vi "Pinholes.vi"(4 "Current Threshold [nA]":dbl, 5 "settling\ndelay":i32) -> (1 "excluded channels":i32[](array[numeric]), 2 "Current [nA]":dbl[](array[numeric]), 3 "Flag":i32[](array[numeric]))   [LabVIEW 2018]
uses:
  general_VIs/globals/QC_MeasurementSetup.vi
  InstrControl/Switching/Switching.lvclass
  InstrControl/SupplyControl/SupplyControl.lvclass
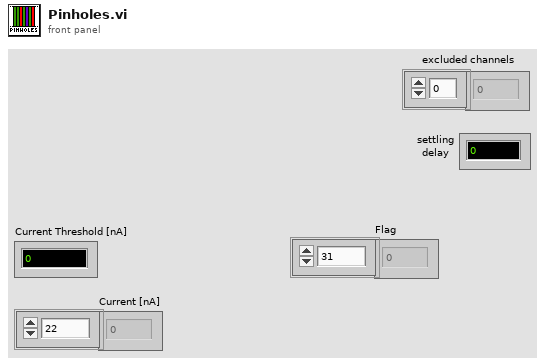
[diagram p1: front panel]
types:
  T1 = cluster{"Bias Supply":refnum<class "SupplyControl.lvclass">, "SMU":refnum<class "SupplyControl.lvclass">, "LCR":refnum<class "LCRControl.lvclass">, "Probe Card Channels":i32, "Bias Voltage [V]":dbl, "First strip":i32, "Last strip":i32, "Base Voltage [V]":dbl, "Base Ramp Step [V]":dbl, "Base Ramp Interval [ms]":u32, "High Voltage [V]":dbl, "High Ramp Step [V]":dbl, "High Ramp Interval [ms]":u32, "Single Needle":bool, "Temperature Readout":enum16{"Read Arduino", "Enter manually"}, "Arduino":refnum<class "ArduinoControl.lvclass">, "Fraction of good strips [%]":dbl, "ProbeStation":refnum<class "ProbeStationControl.lvclass">, "AC frequency [Hz]":i32, "Switching":refnum<class "Switching.lvclass">, "Matrix used?":bool, "Matrix X Channels":cluster{"Bias Supply / SMU LO":i32, "Bias Supply / SMU HI":i32, "CV Box LO":i32, "CV Box HI":i32, "CV Box LO IN":i32, "CV Box HI IN":i32, "Volt meter LO":i32, "Volt meter HI":i32, "Mux1 C1":i32, "Mux1 C2":i32, "Mux2 C1":i32, "Mux2 C2":i32}, "Pinholes Y/N":bool, "Capacitance Y/N":bool, "Resistance Y/N":bool}
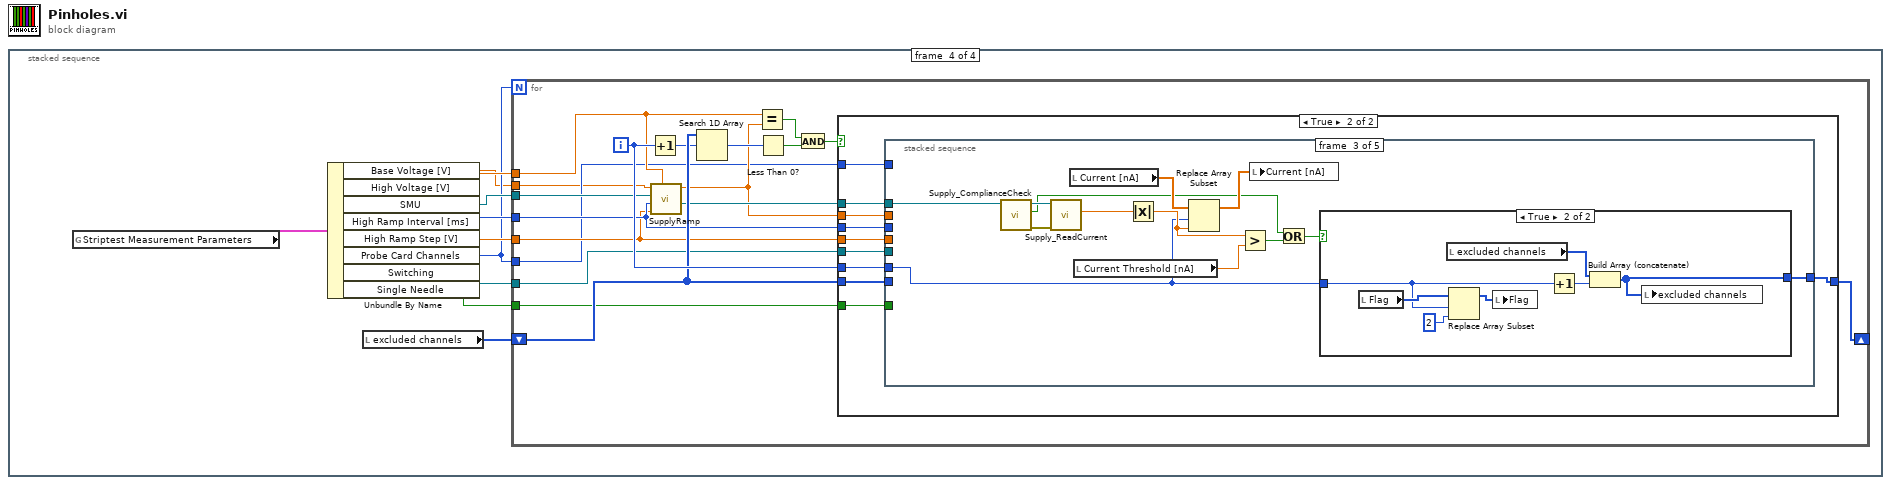
[diagram p0: block diagram]
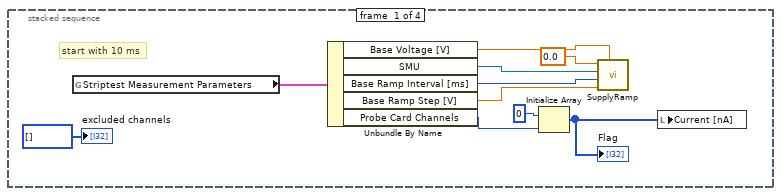
[diagram p2: hidden frame]
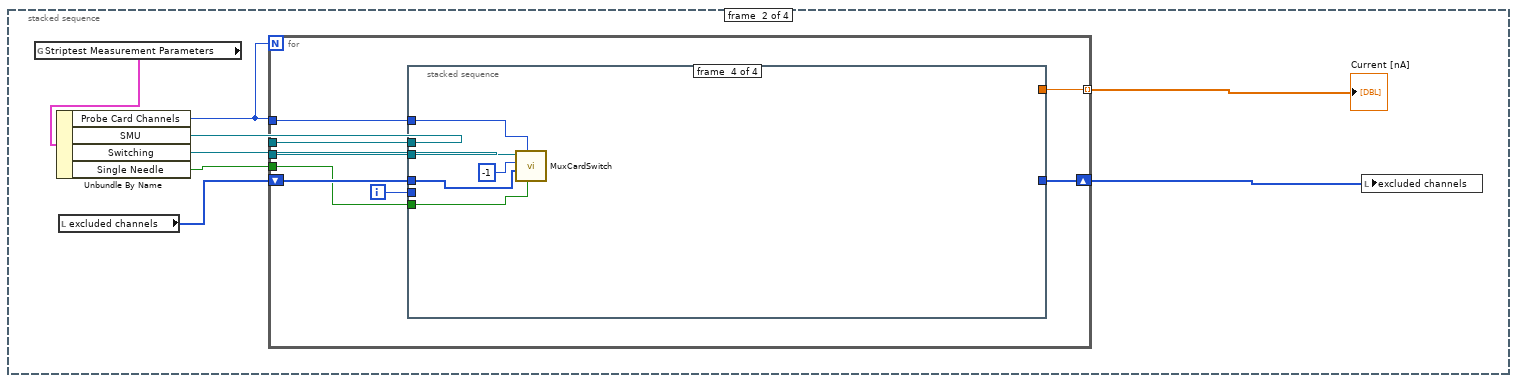
[diagram p3: hidden frame]
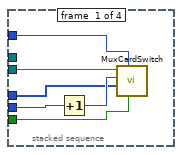
[diagram p4: hidden frame]
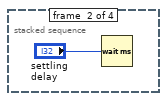
[diagram p5: hidden frame]
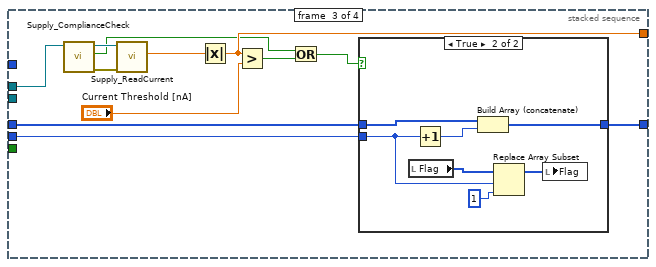
[diagram p6: hidden frame]
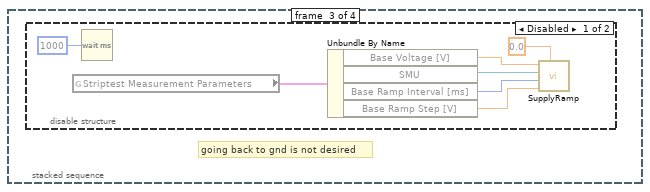
[diagram p8: hidden frame]
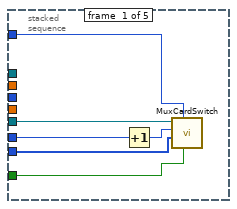
[diagram p11: hidden frame]
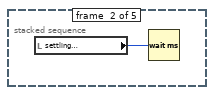
[diagram p12: hidden frame]
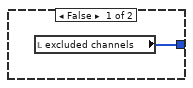
[diagram p13: hidden frame]
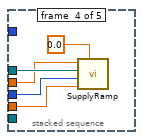
[diagram p14: hidden frame]
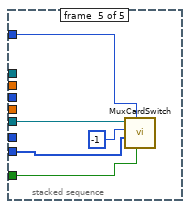
[diagram p15: hidden frame]
diagram:
  n1 = stacked-sequence {
    frame #0 {
      # "start with 10 ms"
      n2 = global read "QC_MeasurementSetup.vi" "Striptest Measurement Parameters"() -> (w6:T1)
      n3 = Unbundle By Name(w6) -> ("Base Voltage [V]"=w5:dbl, "SMU"=w1:refnum<class "SupplyControl.lvclass">, "Base Ramp Interval [ms]"=w4:u32, "Base Ramp Step [V]"=w3:dbl, "Probe Card Channels"=w2:i32)
      n4 = Initialize Array(0, w2) -> (w7:i32[])
      "Flag" <- w7
      n5 = call "SupplyRamp.vi"("Requested Voltage"=w5, "Step Size"=w3, "Step Delay"=w4, "Supply IN"=w1, "Starting Voltage"=0.0) -> ()  [unwired: 3 in, 4 out]
      n6 = local write "Current [nA]"(w7) -> ()
      "excluded channels" <- i32[] []
    }
    frame #1 {
      n7 = global read "QC_MeasurementSetup.vi" "Striptest Measurement Parameters"() -> (w16:T1)
      n8 = Unbundle By Name(w16) -> ("Probe Card Channels"=w11:i32, "SMU"=w15:refnum<class "SupplyControl.lvclass">, "Switching"=w13:refnum<class "Switching.lvclass">, "Single Needle"=w12:bool)
      n9 = local read "excluded channels"() -> (w17:i32[])
      n10 = for {
        N: w11 -> [_]
        tunnel: w11 -> [w26]
        tunnel: [w25] -> w18 mode=indexing
        shift-right: [w22] -> w14
        shift-left: w17 -> [w24]
        tunnel: w13 -> [w19]
        tunnel: w12 -> [w21]
        tunnel: w15 -> [w20]
        i -> [w23]
        n11 = stacked-sequence {
          tunnel: w23 -> [w29 _ w34 _]
          tunnel: w26 -> [w31 _ _ w55]
          tunnel: w24 -> [w30 _ w36 w54]
          tunnel: [_ _ w41 _] -> w25
          tunnel: [_ _ w42 _] -> w22
          tunnel: w19 -> [w28 _ _ w57]
          tunnel: w21 -> [w27 _ _ w56]
          tunnel: w20 -> [_ _ w35 _]
          frame #0 {
            n12 = Increment(x=w29) -> (x+1=w32:i32)
            n13 = call-dynamic "MuxCardSwitch.vi"("Single Needle"=w27, "Probe Card Channels"=w31, "disabled channels"=w30, "Switch to channel"=w32, "Switching in"=w28) -> ()  [unwired: 4 in, 3 out]
          }
          frame #1 {
            n14 = Wait (ms)(milliseconds to wait="settling\ndelay") -> ()  [unwired: 1 out]
          }
          frame #2 {
            n15 = call-dynamic "Supply_ComplianceCheck.vi"("SupplyControl in"=w35) -> ("error out"=w40:errorcluster, "Compliance exceeded?"=w37:bool, "SupplyControl out"=w39:refnum<class "SupplyControl.lvclass">)  [unwired: 7 in, 1 out]
            n16 = call-dynamic "Supply_ReadCurrent.vi"("error in (no error)"=w40, "SupplyControl in"=w39) -> ("Current in nA"=w38:dbl)  [unwired: 7 in, 2 out]
            n17 = Absolute Value(x=w38) -> (abs(x)=w41:dbl)
            n18 = Greater?(x=w41, y="Current Threshold [nA]") -> (0:w43:bool)
            n19 = Or(x=w37, y=w43) -> (x .or. y?=w44:bool)
            n20 = case shown="True" w44 {
              tunnel: w36 -> [w46 w47]
              tunnel: [w46 w49] -> w42
              tunnel: w34 -> [_ w48]
              frame False {
              }
              frame True {
                n21 = local read "Flag"() -> (w53:i32[])
                n22 = Increment(x=w48) -> (x+1=w50:i32)
                n23 = Build Array (concatenate)(w47, w50) -> (w49:i32[])
                n24 = Replace Array Subset(array=w53, new element=1, index=w48) -> (w51:i32[])
                n25 = local write "Flag"(w51) -> ()
              }
            }
          }
          frame #3 {
            n26 = call-dynamic "MuxCardSwitch.vi"("Single Needle"=w56, "Probe Card Channels"=w55, "disabled channels"=w54, "Switch to channel"=-1, "Switching in"=w57) -> ()  [unwired: 4 in, 3 out]
          }
        }
      }
      "Current [nA]" <- w18
      n27 = local write "excluded channels"(w14) -> ()
    }
    frame #2 {
      # "going back to gnd is not desired"
      n28 = disable-structure shown="Disabled" {
        frame Disabled {
          n29 = global read "QC_MeasurementSetup.vi" "Striptest Measurement Parameters"() -> (w63:T1)
          n30 = Wait (ms)(milliseconds to wait=1000) -> ()  [unwired: 1 out]
          n31 = Unbundle By Name(w63) -> ("Base Voltage [V]"=w61:dbl, "SMU"=w62:refnum<class "SupplyControl.lvclass">, "Base Ramp Interval [ms]"=w60:u32, "Base Ramp Step [V]"=w59:dbl)
          n32 = call "SupplyRamp.vi"("Requested Voltage"=0.0, "Step Size"=w59, "Step Delay"=w60, "Supply IN"=w62, "Starting Voltage"=w61) -> ()  [unwired: 3 in, 4 out]
        }
        frame Enabled {
        }
      }
    }
    frame #3 {
      n33 = global read "QC_MeasurementSetup.vi" "Striptest Measurement Parameters"() -> (w74:T1)
      n34 = Unbundle By Name(w74) -> ("Base Voltage [V]"=w66:dbl, "High Voltage [V]"=w73:dbl, "SMU"=w72:refnum<class "SupplyControl.lvclass">, "High Ramp Interval [ms]"=w71:u32, "High Ramp Step [V]"=w70:dbl, "Probe Card Channels"=w68:i32, "Switching"=w69:refnum<class "Switching.lvclass">, "Single Needle"=w67:bool)
      n35 = local read "excluded channels"() -> (w75:i32[])
      n36 = for {
        N: w68 -> [_]
        shift-right: [w93] -> _
        shift-left: w75 -> [w91]
        tunnel: w73 -> [w83]
        tunnel: w72 -> [w82]
        tunnel: w71 -> [w81]
        tunnel: w70 -> [w80]
        tunnel: w69 -> [w79]
        tunnel: w68 -> [w78]
        tunnel: w67 -> [w77]
        tunnel: w66 -> [w76]
        i -> [w92]
        n37 = Increment(x=w92) -> (x+1=w90:i32)
        n38 = call "SupplyRamp.vi"("Requested Voltage"=w83, "Step Size"=w80, "Step Delay"=w81, "Supply IN"=w82, "Starting Voltage"=w76) -> ("Supply OUT"=w85:refnum<class "SupplyControl.lvclass">, "Current Voltage"=w84:dbl)  [unwired: 3 in, 2 out]
        n39 = Search 1D Array(1D array=w91, element=w90) -> (index of element=w89:i32)  [unwired: 1 in]
        n40 = Equal?(x=w83, y=w84) -> (x = y?=w86:bool)
        n41 = Less Than 0?(x=w89) -> (x < 0?=w88:bool)
        n42 = And(x=w86, y=w88) -> (x .and. y?=w87:bool)
        n43 = case shown="True" w87 {
          tunnel: w91 -> [w94 w104]
          tunnel: w92 -> [_ w103]
          tunnel: [w94 w102] -> w93
          tunnel: w80 -> [_ w101]
          tunnel: w78 -> [_ w100]
          tunnel: w79 -> [_ w99]
          tunnel: w77 -> [_ w98]
          tunnel: w85 -> [_ w97]
          tunnel: w84 -> [_ w96]
          tunnel: w81 -> [_ w95]
          frame False {
          }
          frame True {
            n44 = stacked-sequence {
              tunnel: w103 -> [w108 _ w112 _ _]
              tunnel: w104 -> [w109 _ _ _ w138]
              tunnel: [_ _ w122 _ _] -> w102
              tunnel: w101 -> [_ _ _ w133 _]
              tunnel: w100 -> [w107 _ _ _ w139]
              tunnel: w99 -> [w106 _ _ _ w141]
              tunnel: w98 -> [w105 _ _ _ w140]
              tunnel: w97 -> [_ _ w114 w136 _]
              tunnel: w96 -> [_ _ _ w135 _]
              tunnel: w95 -> [_ _ _ w134 _]
              frame #0 {
                n45 = Increment(x=w108) -> (x+1=w110:i32)
                n46 = call-dynamic "MuxCardSwitch.vi"("Single Needle"=w105, "Probe Card Channels"=w107, "disabled channels"=w109, "Switch to channel"=w110, "Switching in"=w106) -> ()  [unwired: 4 in, 3 out]
              }
              frame #1 {
                n47 = local read "settling\ndelay"() -> (w111:i32)
                n48 = Wait (ms)(milliseconds to wait=w111) -> ()  [unwired: 1 out]
              }
              frame #2 {
                n49 = call-dynamic "Supply_ComplianceCheck.vi"("SupplyControl in"=w114) -> ("error out"=w116:errorcluster, "Compliance exceeded?"=w113:bool, "SupplyControl out"=w117:refnum<class "SupplyControl.lvclass">)  [unwired: 7 in, 1 out]
                n50 = call-dynamic "Supply_ReadCurrent.vi"("error in (no error)"=w116, "SupplyControl in"=w117) -> ("Current in nA"=w115:dbl)  [unwired: 7 in, 2 out]
                n51 = local read "Current [nA]"() -> (w119:dbl[])
                n52 = local read "Current Threshold [nA]"() -> (w121:dbl)
                n53 = Absolute Value(x=w115) -> (abs(x)=w118:dbl)
                n54 = Replace Array Subset(array=w119, new element=w118, index=w112) -> (w120:dbl[])
                n55 = Greater?(x=w118, y=w121) -> (0:w123:bool)
                n56 = local write "Current [nA]"(w120) -> ()
                n57 = Or(x=w113, y=w123) -> (x .or. y?=w124:bool)
                n58 = case shown="True" w124 {
                  tunnel: w112 -> [_ w128]
                  tunnel: [w125 w126] -> w122
                  frame False {
                    n59 = local read "excluded channels"() -> (w125:i32[])
                  }
                  frame True {
                    n60 = local read "Flag"() -> (w132:i32[])
                    n61 = local read "excluded channels"() -> (w129:i32[])
                    n62 = Replace Array Subset(array=w132, new element=2, index=w128) -> (w130:i32[])
                    n63 = local write "Flag"(w130) -> ()
                    n64 = Increment(x=w128) -> (x+1=w127:i32)
                    n65 = Build Array (concatenate)(w129, w127) -> (w126:i32[])
                    n66 = local write "excluded channels"(w126) -> ()
                  }
                }
              }
              frame #3 {
                n67 = call "SupplyRamp.vi"("Requested Voltage"=0.0, "Step Size"=w133, "Step Delay"=w134, "Supply IN"=w136, "Starting Voltage"=w135) -> ()  [unwired: 3 in, 4 out]
              }
              frame #4 {
                n68 = call-dynamic "MuxCardSwitch.vi"("Single Needle"=w140, "Probe Card Channels"=w139, "disabled channels"=w138, "Switch to channel"=-1, "Switching in"=w141) -> ()  [unwired: 4 in, 3 out]
              }
            }
          }
        }
      }
    }
  }
